vi "Build Test EXE.vi"() -> ()   [LabVIEW 2019]
uses:
  <vilib>/AppBuilder/AB_API_Simple/Build Specification Version.ctl
  <vilib>/AppBuilder/AB_API_Simple/Set Build Specification Version (path).vi
  <vilib>/AppBuilder/AB_API_Simple/Build (path).vi
  <vilib>/AppBuilder/AB_API_Simple/NI_App_Builder_API.lvlib
panel:
  in  "Build Specification Version":T1={"Major"=2, "Minor"=0, "Fix"=0, "Build"=0}
  in  "Name of build specification (if empty: clean all)":string="Test EXE"
  in  "Path to project":path=path "C:/user/patrick/git/Multichannel-Lockin/src/Multichannel Lockin.lvproj"
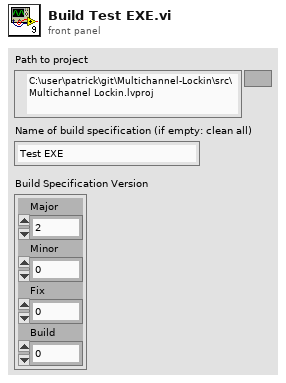
[diagram p1: front panel]
types:
  T1 = typedef "NI_App_Builder_API.lvlib/Build Specification Version.ctl" = cluster{"Major":u16, "Minor":u16, "Fix":u16, "Build":u16}
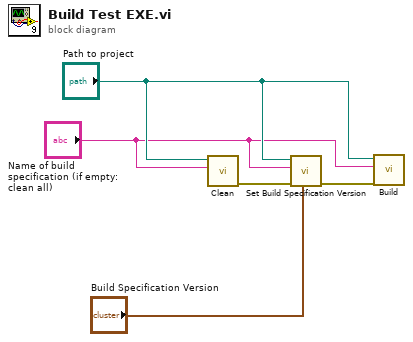
[diagram p0: block diagram]
diagram:
  n1 = call <vilib>:"Clean.vi"("Name of build specification (if empty: clean all)"="Name of build specification (if empty: clean all)", "Path to project"="Path to project") -> ("error out"=w4:errorcluster)  [unwired: 9 in]
  n2 = call-poly <vilib>:"Set Build Specification Version.vi"("Build Specification Version"="Build Specification Version", "error in (no error)"=w4, "Name of build specification"="Name of build specification (if empty: clean all)", "Path to project"="Path to project") -> ("error out"=w3:errorcluster)  [unwired: 7 in]
  n3 = call-poly <vilib>:"Build.vi"("error in (no error)"=w3, "Name of build specification (if empty: build all)"="Name of build specification (if empty: clean all)", "Path to project"="Path to project") -> ()  [unwired: 7 in, 2 out]
